vi "SetDataSetId.vi"(7 "DataSetType":T1, 9 "DataSetName":string, 10 "DataSetIds":variant, 11 "props in":T2[](array[typedef])) -> (3 "props out":T2[](array[typedef]))   [LabVIEW 2017, in "DataEventCreator.lvlib"]
uses:
  <vilib>/addons/InsightCM/Devices/Shared/Common/DataEventCreator/DataEventCreator.lvlib
  <vilib>/addons/InsightCM/MessageBus/Base/controls/KeyValuePair.ctl
  <vilib>/addons/InsightCM/Devices/Shared/Common/DataEvent/controls/DataSetType.ctl
  <vilib>/addons/InsightCM/Utilities/PropertyHelpers/PropertyHelpers.lvlib
  <vilib>/addons/InsightCM/Devices/Shared/Common/DataEvent/DataEvent.lvlib
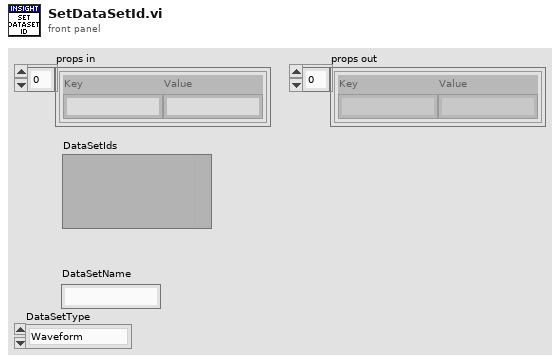
[diagram p1: front panel]
types:
  T1 = typedef "DataEvent.lvlib/DataSetType.ctl" = enum16{"Waveform", "SpeedProfile", "ThermalImage", "EmsaSweep"}
  T2 = typedef "KeyValuePair.ctl" = cluster{"Key":string, "Value":string}
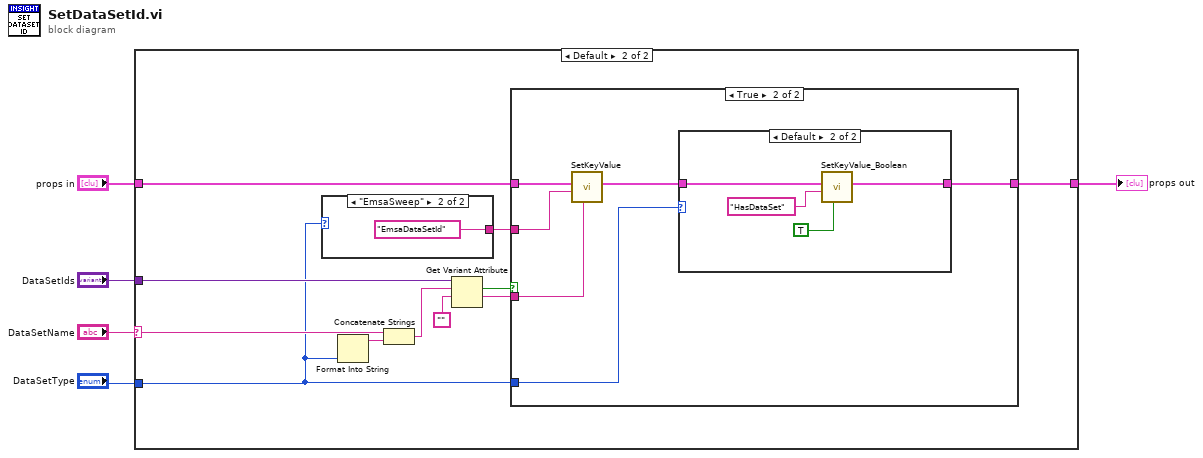
[diagram p0: block diagram]
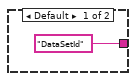
[diagram p3: hidden frame]
diagram:
  n1 = case shown="Default" "DataSetName" {
    selector: "DataSetName" -> [_ w11]
    tunnel: [w6 w8] -> w5
    tunnel: "props in" -> [w6 w15]
    tunnel: "DataSetIds" -> [_ w17]
    tunnel: "DataSetType" -> [_ w7]
    frame "" {
    }
    frame Default {
      n2 = case shown="\"EmsaSweep\"" w7 {
        tunnel: ["DataSetId" "EmsaDataSetId"] -> w14
        frame Default {
        }
        frame "EmsaSweep" {
        }
      }
      n3 = Format Into String(w7) -> (resulting string=w10:string)  [unwired: 3 in, 1 out]
      n4 = Concatenate Strings(w11, w10) -> (w9:string)
      n5 = Get Variant Attribute(Variant=w17, name=w9, default value (empty Variant)="") -> (found=w12:bool, value=w13:string)  [unwired: 1 in, 2 out]
      n6 = case shown="True" w12 {
        tunnel: w15 -> [w20 w26]
        tunnel: [w20 w22] -> w8
        tunnel: w14 -> [_ w25]
        tunnel: w13 -> [_ w24]
        tunnel: w7 -> [_ w21]
        frame False {
        }
        frame True {
          n7 = call <vilib>:"SetKeyValue.vi"("value"=w24, "key"=w25, "key value pairs"=w26) -> ("key value pairs out"=w23:T2[])  [unwired: 8 in]
          n8 = case shown="Default" w21 {
            tunnel: [w27 w28] -> w22
            tunnel: w23 -> [w27 w29]
            frame "Waveform", "SpeedProfile" {
            }
            frame Default {
              n9 = call <vilib>:"SetKeyValue_Boolean.vi"("value"=TRUE, "key"="HasDataSet", "key value pairs"=w29) -> ("key value pairs out"=w28:T2[])  [unwired: 8 in]
            }
          }
        }
      }
    }
  }
  "props out" <- w5
